vi "Initialise DVRs.vi"(8 "error in (no error)":errorcluster) -> (0 "error out":errorcluster, 3 "Data":T1)   [LabVIEW 2021, in "BT.lvlib" / "bt_Blackboard.lvclass"]
uses:
  bt_Blackboard.lvclass
  bt_Blackboard.lvclass/bt_Blackboard.ctl
  Status Type.ctl
  Data DVR Type.ctl
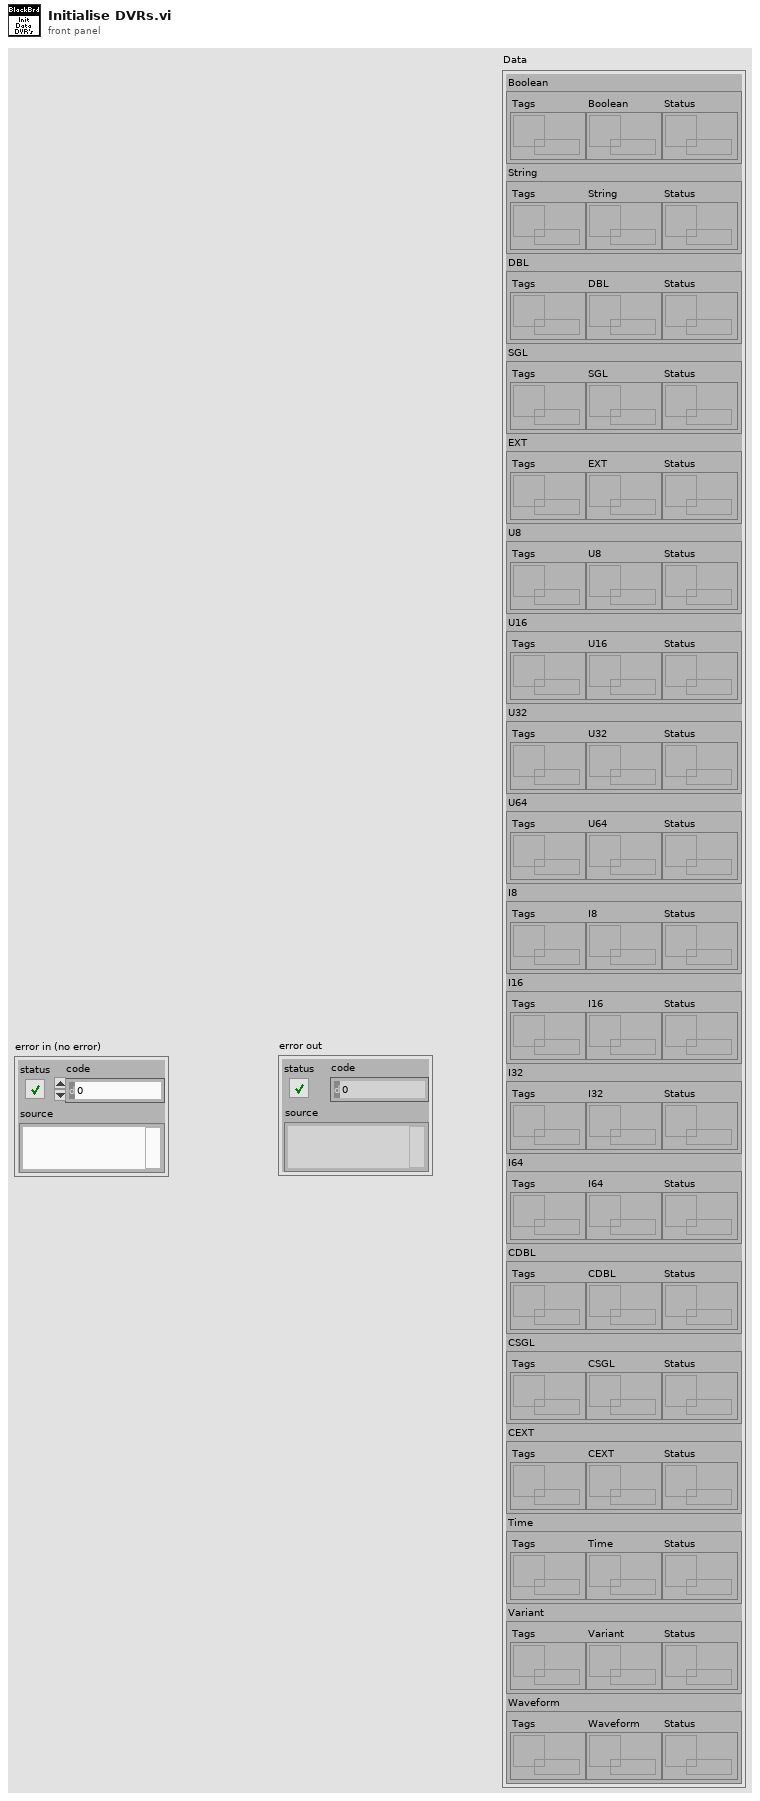
[diagram p1: front panel]
types:
  T1 = typedef "BT.lvlib/bt_Blackboard.lvclass/Data DVR Type.ctl" = cluster{"Boolean":cluster{"Tags":refnum<data-value>, "Boolean":refnum<data-value>, "Status":refnum<data-value>}, "String":cluster{"Tags":refnum<data-value>, "String":refnum<data-value>, "Status":refnum<data-value>}, "DBL":cluster{"Tags":refnum<data-value>, "DBL":refnum<data-value>, "Status":refnum<data-value>}, "SGL":cluster{"Tags":refnum<data-value>, "SGL":refnum<data-value>, "Status":refnum<data-value>}, "EXT":cluster{"Tags":refnum<data-value>, "EXT":refnum<data-value>, "Status":refnum<data-value>}, "U8":cluster{"Tags":refnum<data-value>, "U8":refnum<data-value>, "Status":refnum<data-value>}, "U16":cluster{"Tags":refnum<data-value>, "U16":refnum<data-value>, "Status":refnum<data-value>}, "U32":cluster{"Tags":refnum<data-value>, "U32":refnum<data-value>, "Status":refnum<data-value>}, "U64":cluster{"Tags":refnum<data-value>, "U64":refnum<data-value>, "Status":refnum<data-value>}, "I8":cluster{"Tags":refnum<data-value>, "I8":refnum<data-value>, "Status":refnum<data-value>}, "I16":cluster{"Tags":refnum<data-value>, "I16":refnum<data-value>, "Status":refnum<data-value>}, "I32":cluster{"Tags":refnum<data-value>, "I32":refnum<data-value>, "Status":refnum<data-value>}, "I64":cluster{"Tags":refnum<data-value>, "I64":refnum<data-value>, "Status":refnum<data-value>}, "CDBL":cluster{"Tags":refnum<data-value>, "CDBL":refnum<data-value>, "Status":refnum<data-value>}, "CSGL":cluster{"Tags":refnum<data-value>, "CSGL":refnum<data-value>, "Status":refnum<data-value>}, "CEXT":cluster{"Tags":refnum<data-value>, "CEXT":refnum<data-value>, "Status":refnum<data-value>}, "Time":cluster{"Tags":refnum<data-value>, "Time":refnum<data-value>, "Status":refnum<data-value>}, "Variant":cluster{"Tags":refnum<data-value>, "Variant":refnum<data-value>, "Status":refnum<data-value>}, "Waveform":cluster{"Tags":refnum<data-value>, "Waveform":refnum<data-value>, "Status":refnum<data-value>}}
  T2 = cluster{"Tags":refnum<data-value>, "Boolean":refnum<data-value>, "Status":refnum<data-value>}
  T3 = cluster{"Tags":refnum<data-value>, "String":refnum<data-value>, "Status":refnum<data-value>}
  T4 = cluster{"Tags":refnum<data-value>, "DBL":refnum<data-value>, "Status":refnum<data-value>}
  T5 = cluster{"Tags":refnum<data-value>, "SGL":refnum<data-value>, "Status":refnum<data-value>}
  T6 = cluster{"Tags":refnum<data-value>, "EXT":refnum<data-value>, "Status":refnum<data-value>}
  T7 = cluster{"Tags":refnum<data-value>, "U8":refnum<data-value>, "Status":refnum<data-value>}
  T8 = cluster{"Tags":refnum<data-value>, "U16":refnum<data-value>, "Status":refnum<data-value>}
  T9 = cluster{"Tags":refnum<data-value>, "U32":refnum<data-value>, "Status":refnum<data-value>}
  T10 = cluster{"Tags":refnum<data-value>, "U64":refnum<data-value>, "Status":refnum<data-value>}
  T11 = cluster{"Tags":refnum<data-value>, "I8":refnum<data-value>, "Status":refnum<data-value>}
  T12 = cluster{"Tags":refnum<data-value>, "I16":refnum<data-value>, "Status":refnum<data-value>}
  T13 = cluster{"Tags":refnum<data-value>, "I32":refnum<data-value>, "Status":refnum<data-value>}
  T14 = cluster{"Tags":refnum<data-value>, "I64 ":refnum<data-value>, "Status":refnum<data-value>}
  T15 = cluster{"Tags":refnum<data-value>, "CDBL":refnum<data-value>, "Status":refnum<data-value>}
  T16 = cluster{"Tags":refnum<data-value>, "CSGL":refnum<data-value>, "Status":refnum<data-value>}
  T17 = cluster{"Tags":refnum<data-value>, "CEXT":refnum<data-value>, "Status":refnum<data-value>}
  T18 = cluster{"Tags":refnum<data-value>, "Time":refnum<data-value>, "Status":refnum<data-value>}
  T19 = cluster{"Tags":refnum<data-value>, "Variant":refnum<data-value>, "Status":refnum<data-value>}
  T20 = cluster{"Tags":refnum<data-value>, "Waveform":refnum<data-value>, "Status":refnum<data-value>}
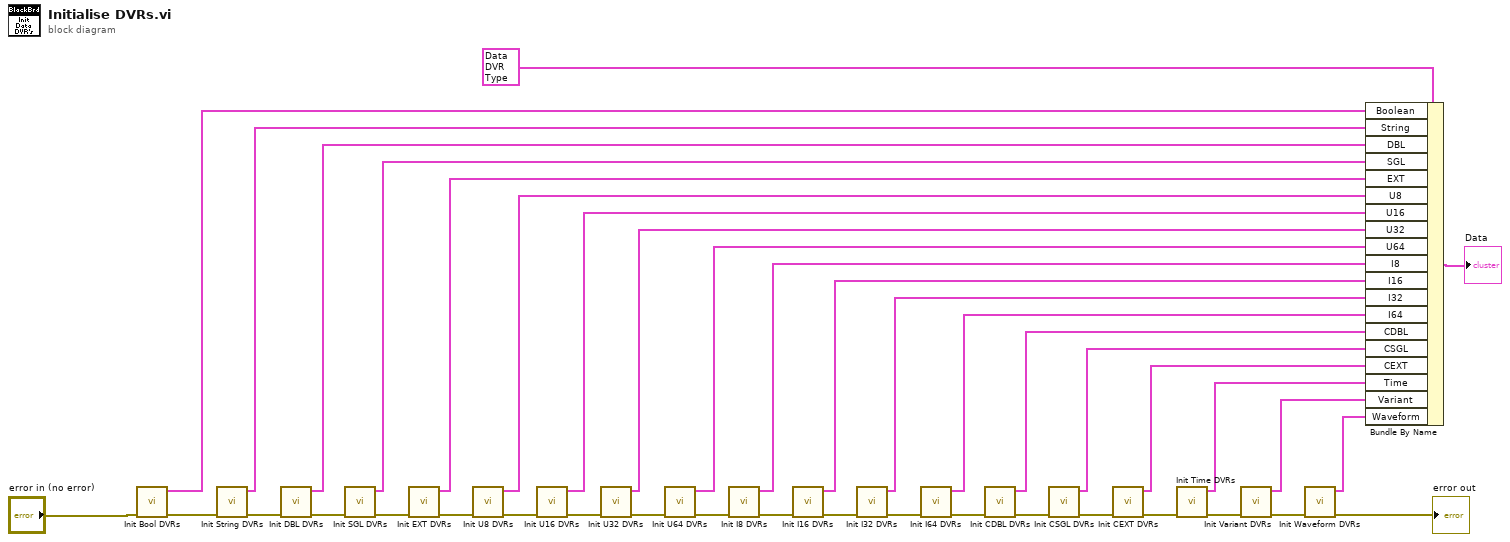
[diagram p0: block diagram]
diagram:
  n1 = call "Init Bool DVRs.vi"("error in (no error)"="error in (no error)") -> ("error out"=w37:errorcluster, "Boolean"=w38:T2)  [unwired: 9 in]
  n2 = call "Init String DVRs.vi"("error in (no error)"=w37) -> ("error out"=w35:errorcluster, "String"=w36:T3)  [unwired: 9 in]
  n3 = call "Init DBL DVRs.vi"("error in (no error)"=w35) -> ("error out"=w33:errorcluster, "DBL"=w34:T4)  [unwired: 9 in]
  n4 = call "Init SGL DVRs.vi"("error in (no error)"=w33) -> ("error out"=w30:errorcluster, "DBL"=w32:T5)  [unwired: 9 in]
  n5 = call "Init EXT DVRs.vi"("error in (no error)"=w30) -> ("error out"=w29:errorcluster, "DBL"=w31:T6)  [unwired: 9 in]
  n6 = call "Init U8 DVRs.vi"("error in (no error)"=w29) -> ("error out"=w27:errorcluster, "U8"=w28:T7)  [unwired: 9 in]
  n7 = call "Init U16 DVRs.vi"("error in (no error)"=w27) -> ("error out"=w25:errorcluster, "U16"=w26:T8)  [unwired: 9 in]
  n8 = call "Init U32 DVRs.vi"("error in (no error)"=w25) -> ("error out"=w23:errorcluster, "U32"=w24:T9)  [unwired: 9 in]
  n9 = call "Init U64 DVRs.vi"("error in (no error)"=w23) -> ("error out"=w21:errorcluster, "U64"=w22:T10)  [unwired: 9 in]
  n10 = call "Init I8 DVRs.vi"("error in (no error)"=w21) -> ("error out"=w19:errorcluster, "I8"=w20:T11)  [unwired: 9 in]
  n11 = call "Init I16 DVRs.vi"("error in (no error)"=w19) -> ("error out"=w17:errorcluster, "I16"=w18:T12)  [unwired: 9 in]
  n12 = call "Init I32 DVRs.vi"("error in (no error)"=w17) -> ("error out"=w15:errorcluster, "I32"=w16:T13)  [unwired: 9 in]
  n13 = call "Init I64 DVRs.vi"("error in (no error)"=w15) -> ("error out"=w13:errorcluster, "I64"=w14:T14)  [unwired: 9 in]
  n14 = call "Init CDBL DVRs.vi"("error in (no error)"=w13) -> ("error out"=w11:errorcluster, "CDBL"=w12:T15)  [unwired: 9 in]
  n15 = call "Init CSGL DVRs.vi"("error in (no error)"=w11) -> ("error out"=w8:errorcluster, "CDBL"=w10:T16)  [unwired: 9 in]
  n16 = call "Init CEXT DVRs.vi"("error in (no error)"=w8) -> ("error out"=w7:errorcluster, "CEXT"=w9:T17)  [unwired: 9 in]
  n17 = call "Init Time DVRs.vi"("error in (no error)"=w7) -> ("error out"=w4:errorcluster, "Time"=w6:T18)  [unwired: 9 in]
  n18 = call "Init Variant DVRs.vi"("error in (no error)"=w4) -> ("error out"=w2:errorcluster, "Variant"=w5:T19)  [unwired: 9 in]
  n19 = call "Init Waveform DVRs.vi"("error in (no error)"=w2) -> ("error out"=→"error out":errorcluster, "Waveform"=w3:T20)  [unwired: 9 in]
  n20 = Bundle By Name(cluster=T1 {"Boolean"={"Tags"=refnum, "Boolean"=refnum, "Status"=refnum}, "String"={"Tags"=refnum, "String"=refnum, "Status"=refnum}, "DBL"={"Tags"=refnum, "DBL"=refnum, "Status"=refnum}, "SGL"={"Tags"=refnum, "SGL"=refnum, "Status"=refnum}, "EXT"={"Tags"=refnum, "EXT"=refnum, "Status"=refnum}, "U8"={"Tags"=refnum, "U8"=refnum, "Status"=refnum}, "U16"={"Tags"=refnum, "U16"=refnum, "Status"=refnum}, "U32"={"Tags"=refnum, "U32"=refnum, "Status"=refnum}, "U64"={"Tags"=refnum, "U64"=refnum, "Status"=refnum}, "I8"={"Tags"=refnum, "I8"=refnum, "Status"=refnum}, "I16"={"Tags"=refnum, "I16"=refnum, "Status"=refnum}, "I32"={"Tags"=refnum, "I32"=refnum, "Status"=refnum}, "I64"={"Tags"=refnum, "I64"=refnum, "Status"=refnum}, "CDBL"={"Tags"=refnum, "CDBL"=refnum, "Status"=refnum}, "CSGL"={"Tags"=refnum, "CSGL"=refnum, "Status"=refnum}, "CEXT"={"Tags"=refnum, "CEXT"=refnum, "Status"=refnum}, "Time"={"Tags"=refnum, "Time"=refnum, "Status"=refnum}, "Variant"={"Tags"=refnum, "Variant"=refnum, "Status"=refnum}, "Waveform"={"Tags"=refnum, "Waveform"=refnum, "Status"=refnum}} ("Data"), "Boolean"=w38, "String"=w36, "DBL"=w34, "SGL"=w32, "EXT"=w31, "U8"=w28, "U16"=w26, "U32"=w24, "U64"=w22, "I8"=w20, "I16"=w18, "I32"=w16, "I64"=w14, "CDBL"=w12, "CSGL"=w10, "CEXT"=w9, "Time"=w6, "Variant"=w5, "Waveform"=w3) -> (→"Data":T1)
